vi "Write id.vi"(8 "error in (no error)":errorcluster, 10 "id":string, 11 "Update Heater DC MSG in":refnum<class "Update Heater DC MSG.lvclass">) -> (0 "error out":errorcluster, 3 "Update Heater DC MSG out":refnum<class "Update Heater DC MSG.lvclass">)   [LabVIEW 2017, in "Controller.lvlib" / "Update Heater DC MSG.lvclass"]
uses:
  Update Heater DC MSG.lvclass
  Update Heater DC MSG.lvclass/Update Heater DC MSG.ctl
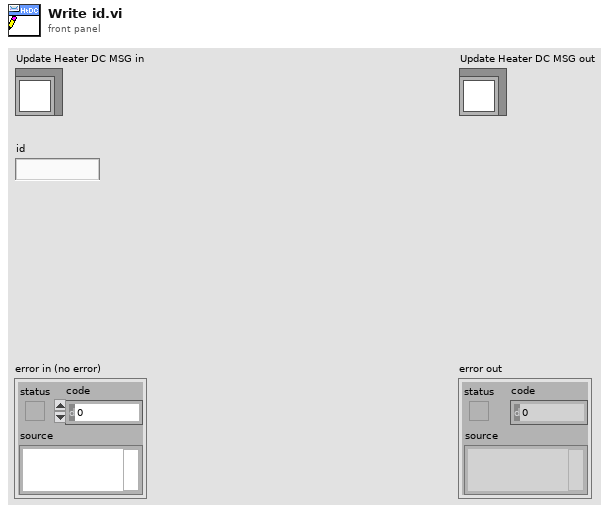
[diagram p1: front panel]
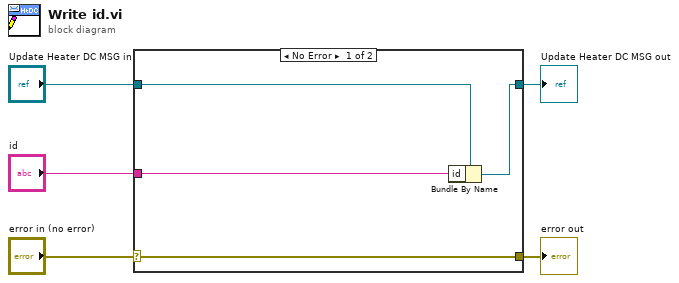
[diagram p0: block diagram]
diagram:
  n1 = case shown="No Error" "error in (no error)" {
    selector: "error in (no error)" -> [w9 w10]
    tunnel: [w9 w10] -> w4
    tunnel: [w7 w11] -> w2
    tunnel: "Update Heater DC MSG in" -> [w8 w11]
    tunnel: "id" -> [w6 _]
    frame No Error {
      n2 = Bundle By Name(cluster=w8, "id"=w6) -> (w7:refnum<class "Update Heater DC MSG.lvclass">)
    }
    frame Error {
    }
  }
  "error out" <- w4
  "Update Heater DC MSG out" <- w2
